vi "Main.vi"(11 "Module Admin":refnum<class "Delacor_lib_QMH_Module Admin.lvclass">) -> ()   [LabVIEW 2021, in "User Interface.lvlib"]
doc: "This template is based off of the Queued Message Handler design pattern and the Queued Message Handler project template that ships with LabVIEW.\n\nThe main difference is that the queue is private to this module and communication between modules is performed via Broadcast and Request events.\n\nRequest events are wrapped in public API methods and are handled in the Event Handling Loop (EHL) of this VI. Any module can register for Broadcast events sent by this module. The EHL generates messages based on user interface actions.\n\nThe Message Handling Loop (MHL) processes messages generated by the EHL, or by other messages. The messages are string values, so new messages can be added easily to the Message Cases case structure in the MHL. Each message cluster can also provide an optional value for Message Data, which is a variant that can be converted to whatever message-specific data is required.\n_____\nBased on DQMH Project Template 6.1.0.94."
uses:
  User Interface.lvlib
  <vilib>/Delacor/Delacor QMH/Libraries/Module Admin_class/Delacor_lib_QMH_Module Admin.lvclass
  Module Data--cluster.ctl
  <vilib>/Delacor/Delacor QMH/Libraries/Message Queue_class/Delacor_lib_QMH_Message Queue.lvclass/Delacor_lib_QMH_Message Queue.ctl
  Stop Argument--cluster.ctl
  <vilib>/Delacor/Delacor QMH/Libraries/Module Admin_class/Delacor_lib_QMH_Module Admin.lvclass/Delacor_lib_QMH_Module Admin.ctl
  REQ UI Title Argument--cluster.ctl
  <vilib>/Utility/miscctls.llb/LVPointTypeDef.ctl
  VI Name.ctl
  <vilib>/Delacor/Delacor QMH/Libraries/Message Queue_class/Delacor_lib_QMH_Enqueue Message (Single).vi
  <vilib>/Delacor/Delacor QMH/Libraries/Module Admin_class/Delacor_lib_QMH_Get External Launch.vi
  <vilib>/Utility/error.llb/Error Cluster From Error Code.vi
  <vilib>/ErrorRing/Error Ring.xnode
  <vilib>/Delacor/Delacor QMH/Libraries/Message Queue_class/Delacor_lib_QMH_Message Queue.lvclass
  Database/Database.lvlib
  CAN/CAN.lvlib
  DAQ Hardware/DAQ Hardware.lvlib
  DAQ IO/DAQ IO.lvlib
  ARINC/ARINC.lvlib
  DC PWS/DC PWS.lvlib
  DMM/DMM.lvlib
  Func Generator/Func Generator.lvlib
  Oscilloscope/Oscilloscope.lvlib
  S-Matrix/S-Matrix.lvlib
  Environment Chamber/Environment Chamber.lvlib
  CVT/CVT.lvlib
panel:
  out "Top Label":string="MAINTENANCE"
  out "Time":string="Sat  8/3/2019  8:10:44 PM"
  out "error out":errorcluster
  out "Status":string
  in  "Simulate MHL Error":bool
  in  "Simulate EHL Error":bool
  # "Other QMH Modules communicate with this Module via its Public API (wrappers for its Request Events).\n\nThis Module communicates with other Modules via its Broadcast Events.\nAny module that wants to get these messages, just registers for this module's Broadcast events."
  # "This template is for the Delacor Modified Queued Message Handler design pattern.\n\nSee the block diagram for more information on how to use this template."
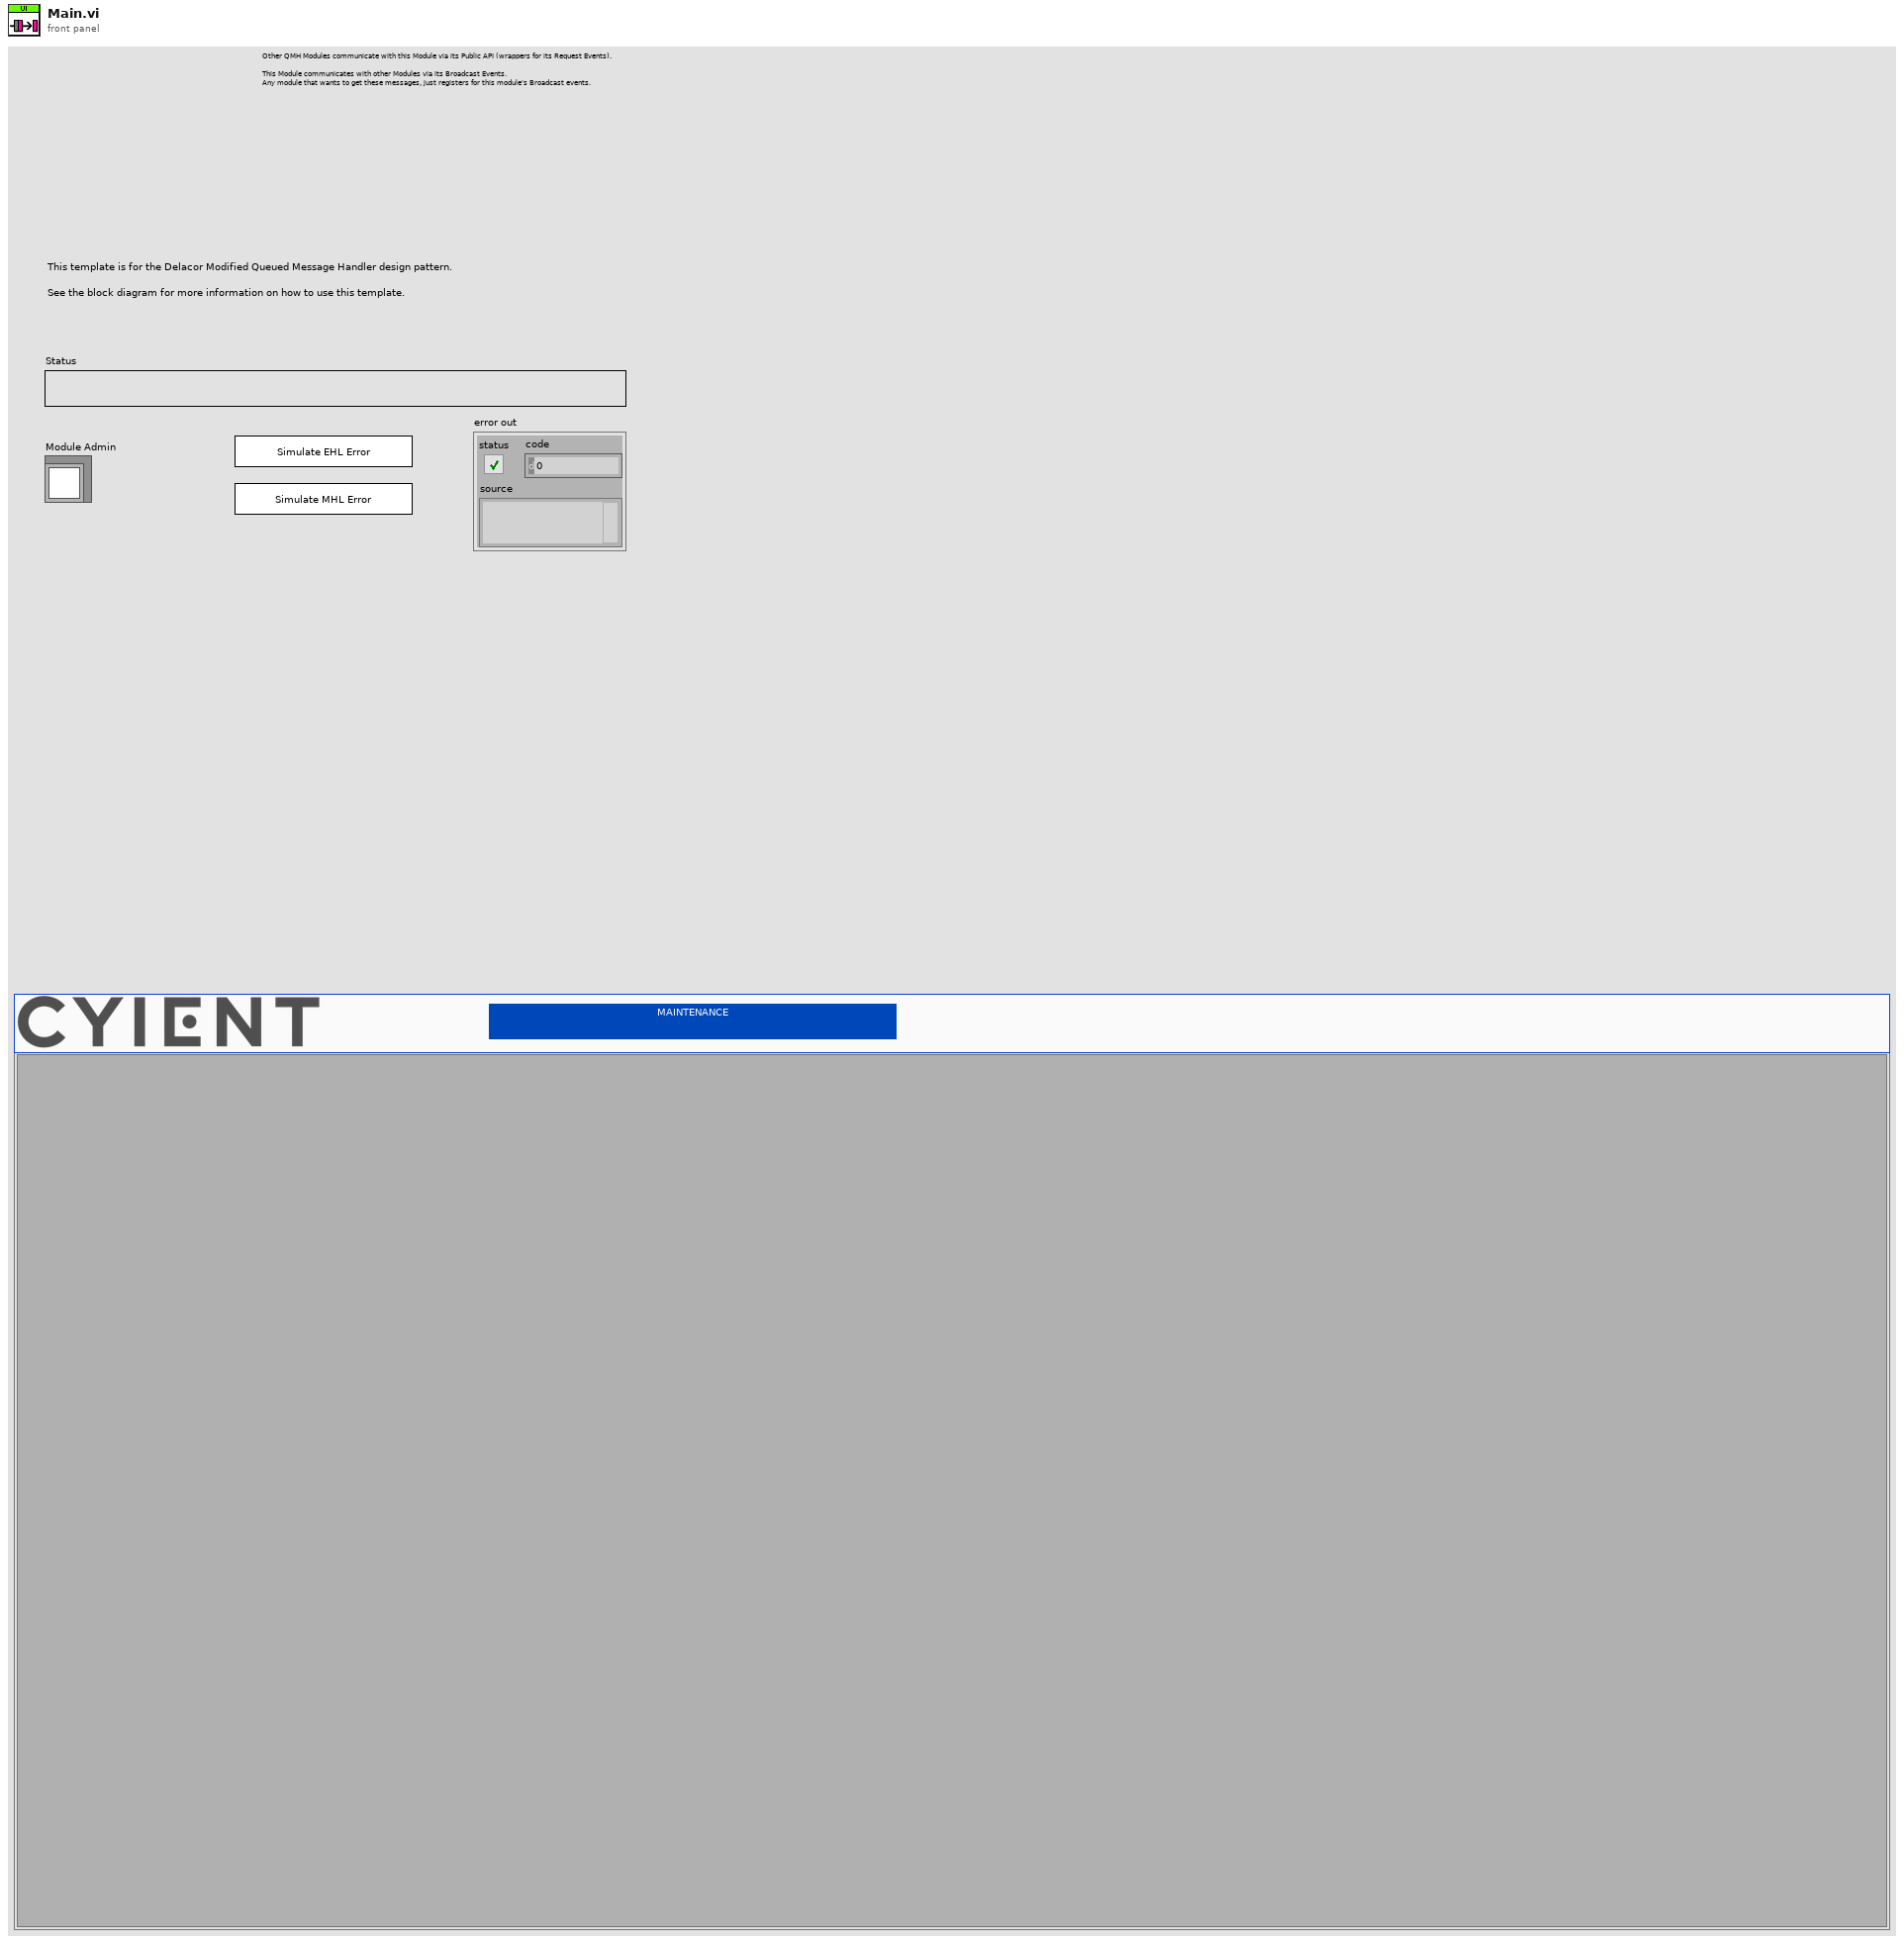
[diagram p1: front panel]
types:
  T1 = typedef "User Interface.lvlib/Request Events--cluster.ctl" = cluster{"Stop Module":refnum<user-event>, "Show Panel":refnum<user-event>, "Hide Panel":refnum<user-event>, "Get Module Execution Status":refnum<user-event>, "Show Diagram":refnum<user-event>, "REQ UI Title":refnum<user-event>}
  T2 = typedef "User Interface.lvlib/Module Data--cluster.ctl" = cluster{"Status":string}
  T3 = enum32{"invalid lock state", "Not Locked", "Locked (No Password)", "Password-protected"}
  T4 = typedef "User Interface.lvlib/Stop Argument--cluster.ctl" = cluster{"Origin":string, "Exit via Stop Module Req?":bool, "Wait for Module to stop?":bool}
  T5 = typedef "User Interface.lvlib/REQ UI Title Argument--cluster.ctl" = cluster{"UI Title":string}
  T6 = typedef "LVPointTypeDef.ctl" = cluster{"Horizontal":i16, "Vertical":i16}
  T7 = enum32{"Invalid", "Standard", "Closed", "Hidden", "Minimized", "Maximized"}
  T8 = typedef "User Interface.lvlib/VI Name.ctl" = enum16{"Dashboard", "Maintenance", "Recipe", "Inst Configuration", "Testing", "Report"}
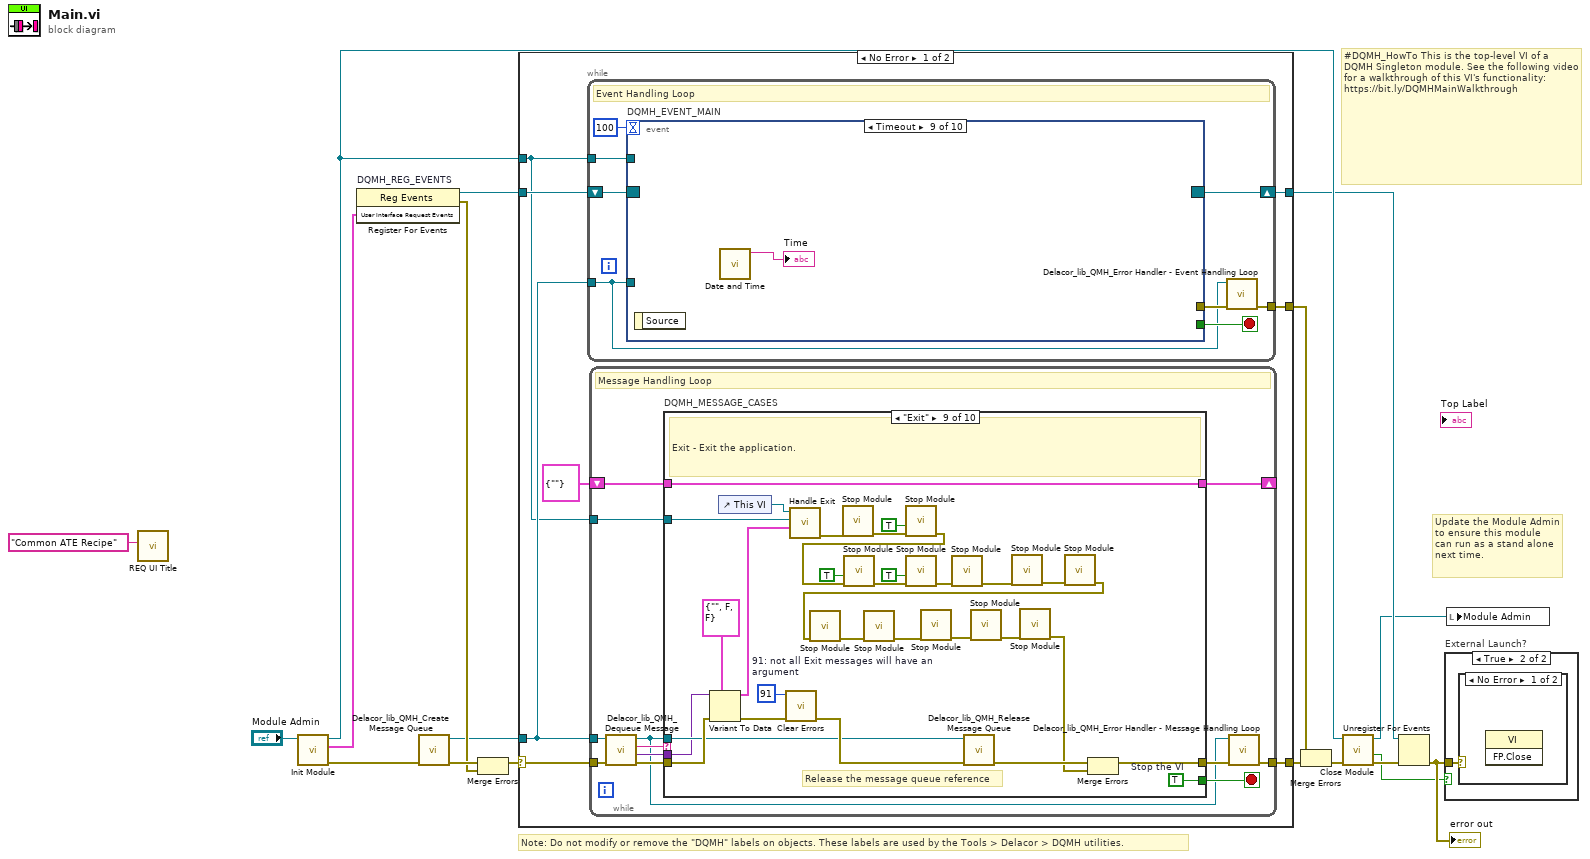
[diagram p0: block diagram]
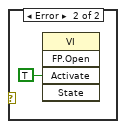
[diagram p3: hidden frame]
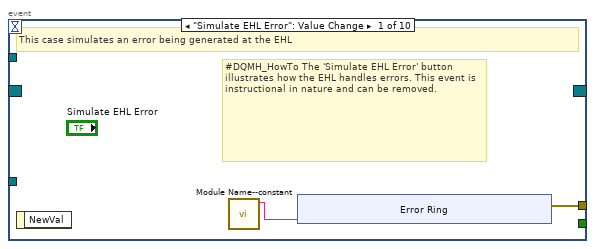
[diagram p4: hidden frame]
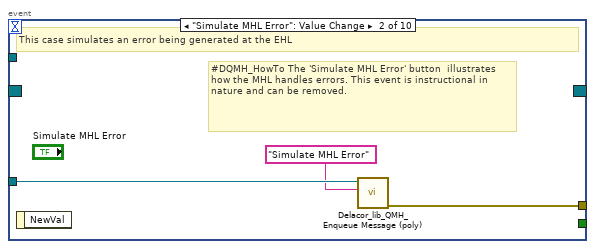
[diagram p5: hidden frame]
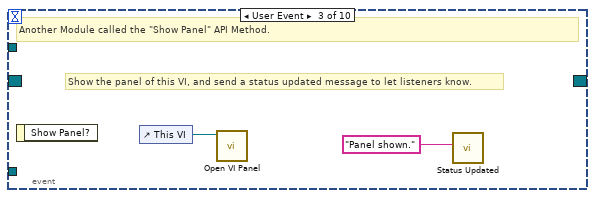
[diagram p6: hidden frame]
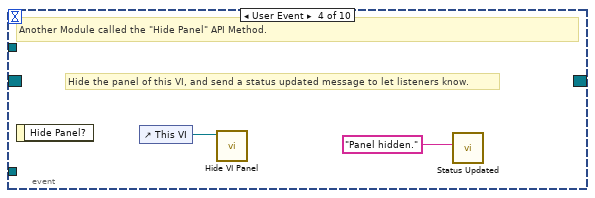
[diagram p7: hidden frame]
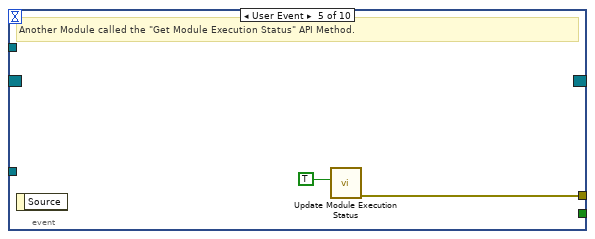
[diagram p8: hidden frame]
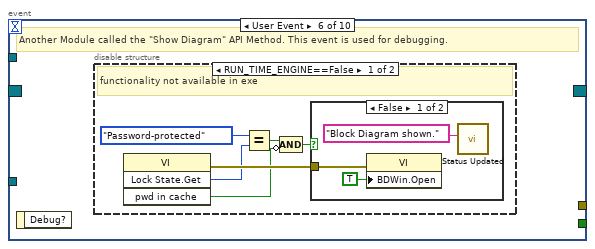
[diagram p9: hidden frame]
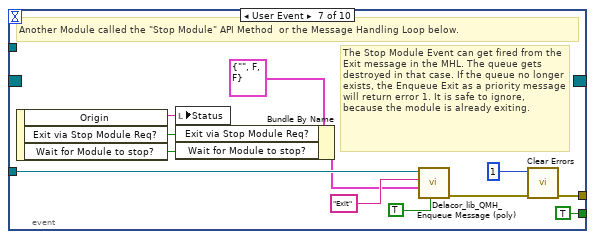
[diagram p12: hidden frame]
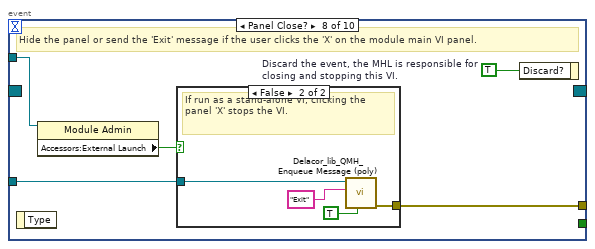
[diagram p13: hidden frame]
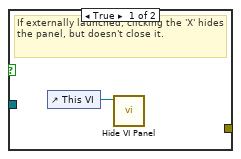
[diagram p14: hidden frame]
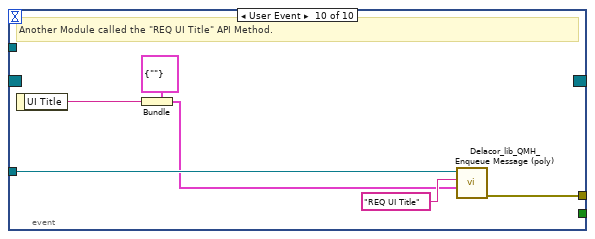
[diagram p15: hidden frame]
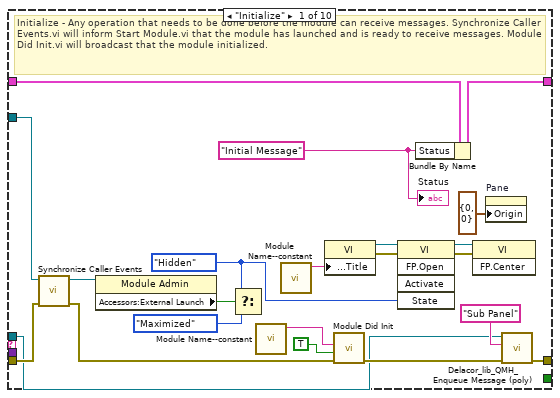
[diagram p16: hidden frame]
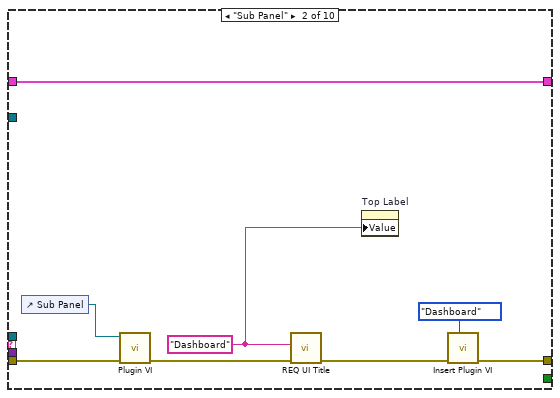
[diagram p17: hidden frame]
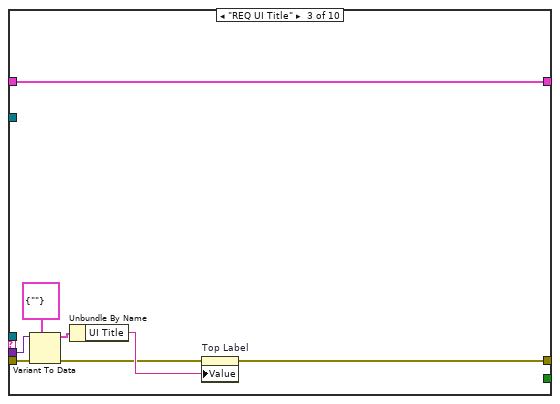
[diagram p18: hidden frame]
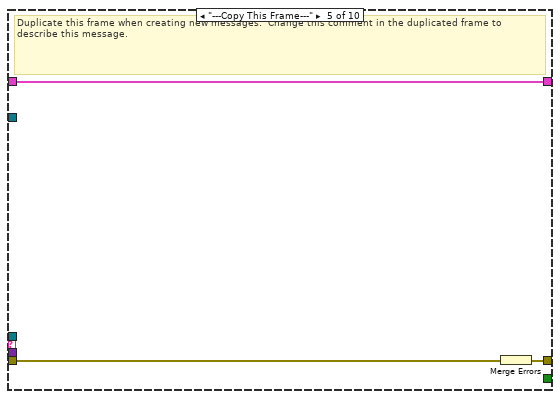
[diagram p20: hidden frame]
diagram:
  # "#DQMH_HowTo This is the top-level VI of a DQMH Singleton module. See the following video for a walkthrough of this VI's functionality: https://bit.ly/DQMHMainWalkthrough"
  # "Note: Do not modify or remove the \"DQMH\" labels on objects. These labels are used by the Tools > Delacor > DQMH utilities."
  # "Update the Module Admin to ensure this module can run as a stand alone next time."
  n1 = call "REQ UI Title.vi"("UI Title"="Common ATE Recipe") -> ()  [unwired: 10 in, 1 out]
  n2 = call "Init Module.vi"("Singleton Module Admin in"="Module Admin") -> ("error out"=w17:errorcluster, "User Interface Request Events"=w6:T1, "Singleton Module Admin out"=w9:refnum<class "Delacor_lib_QMH_Module Admin.lvclass">)  [unwired: 8 in]
  n3 = register-events "DQMH_REG_EVENTS"(w6) -> (reference out=w7:refnum<event-registration>, error out=w10:errorcluster)  [unwired: 2 in]
  n4 = call <vilib>:"Delacor_lib_QMH_Create Message Queue.vi"("error in"=w17) -> ("error out"=w12:errorcluster, "Message Queue"=w5:refnum<class "Delacor_lib_QMH_Message Queue.lvclass">)  [unwired: 9 in]
  n5 = Merge Errors(w12, w10) -> (w11:errorcluster)
  n6 = case shown="No Error" w11 {
    selector: w11 -> [w24 w222]
    tunnel: [w26 w221] -> w18
    tunnel: [w23 w227] -> w8
    tunnel: w7 -> [w21 w227]
    tunnel: w5 -> [w20 w220]
    tunnel: [w25 _] -> w15
    tunnel: w9 -> [w19 w223]
    frame No Error {
      n7 = while {
        tunnel: w20 -> [w28]
        shift-right: [w31] -> w23
        shift-left: w21 -> [w32]
        tunnel: [w33] -> w25
        tunnel: w19 -> [w29]
        stop <- w30 stop-if-true
        # "Event Handling Loop"
        n8 = event "DQMH_EVENT_MAIN" shown="[8] Timeout" {
          selector: w32 -> [_ _ _ _ _ _ _ _ _ _]
          dyn-events: [_ _ _ _ _ _ _ _ _ _] -> w31
          timeout: 100 -> [_ _ _ _ _ _ _ _ _ _]
          tunnel: [_ _ _ _ _ _ TRUE ("Discard?") _ _ _] -> w30
          tunnel: w28 -> [_ w45 _ _ _ _ w69 w76 _ w90]
          tunnel: [w36 w46 _ _ w52 _ w72 w78 _ w85] -> w34
          tunnel: w29 -> [_ _ _ _ _ _ _ w75 _ _]
          event "Simulate EHL Error": Value Change {
            # "#DQMH_HowTo The 'Simulate EHL Error' button  illustrates how the EHL handles errors. This event is instructional in nature and can be removed."
            # "This case simulates an error being generated at the EHL"
            n9 = event-data() -> ()  [unwired: 1 in, 1 out]
            n10 = call "Module Name--constant.vi"() -> ("Module Name"=w35:string)  [unwired: 11 in]
            n11 = xnode "Error Ring"("parameter 0"=w35) -> ("error out"=w36:errorcluster)
          }
          event "Simulate MHL Error": Value Change {
            # "#DQMH_HowTo The 'Simulate MHL Error' button  illustrates how the MHL handles errors. This event is instructional in nature and can be removed."
            # "This case simulates an error being generated at the EHL"
            n12 = event-data() -> ()  [unwired: 1 in, 1 out]
            n13 = call-poly <vilib>:"Delacor_lib_QMH_Enqueue Message (poly).vi"("Message"="Simulate MHL Error", "Message Queue in"=w45) -> ("error out"=w46:errorcluster)  [unwired: 8 in, 1 out]
          }
          event User Event {
            # "Show the panel of this VI, and send a status updated message to let listeners know."
            # "Another Module called the \"Show Panel\" API Method."
            n14 = event-data() -> ()  [unwired: 1 in, 1 out]
            n15 = control-ref of="This VI"() -> (w48:refnum<vi>)
            n16 = call "Open VI Panel.vi"("VI"=w48) -> ()  [unwired: 10 in, 1 out]
            n17 = call "Status Updated.vi"("Status"="Panel shown." ("format string")) -> ()  [unwired: 10 in, 1 out]
          }
          event User Event {
            # "Hide the panel of this VI, and send a status updated message to let listeners know."
            # "Another Module called the \"Hide Panel\" API Method."
            n18 = event-data() -> ()  [unwired: 1 in, 1 out]
            n19 = control-ref of="This VI"() -> (w50:refnum<vi>)
            n20 = call "Hide VI Panel.vi"("VI"=w50) -> ()  [unwired: 10 in, 1 out]
            n21 = call "Status Updated.vi"("Status"="Panel hidden." ("format string")) -> ()  [unwired: 10 in, 1 out]
          }
          event User Event {
            # "Another Module called the \"Get Module Execution Status\" API Method."
            n22 = event-data() -> ()  [unwired: 1 in, 1 out]
            n23 = call "Update Module Execution Status.vi"("Running?"=TRUE) -> ("error out"=w52:errorcluster)  [unwired: 10 in]
          }
          event User Event {
            # "Another Module called the \"Show Diagram\" API Method. This event is used for debugging."
            n24 = event-data() -> ()  [unwired: 1 in, 1 out]
            n25 = disable-structure shown="RUN_TIME_ENGINE==False" {
              frame condition #0 (active) {
                # "functionality not available in exe"
                n26 = invoke class="VI" method="Lock State.Get"() -> (error out=w58:errorcluster, "Get Lock State"=w57:T3, "pwd in cache"=w54:bool)  [unwired: 4 in, 1 out]
                n27 = Equal?(x=T3."Password-protected", y=w57) -> (x = y?=w55:bool)
                n28 = Compound Arithmetic op=AND(w55, invert w54) -> (w53:bool)
                n29 = case shown="False" w53 {
                  tunnel: w58 -> [w61 _]
                  frame False {
                    n30 = property class="VI"(error in=w61, "BDWin.Open"=TRUE ("Block Diagram Window:Open")) -> ()  [unwired: 1 in, 2 out]
                    n31 = call "Status Updated.vi"("Status"="Block Diagram shown." ("format string")) -> ()  [unwired: 10 in, 1 out]
                  }
                  frame True {
                    # "Password-protected VI, and the password is not in the cache. Do not show the diagram."
                  }
                }
              }
              frame condition #1 {
              }
            }
          }
          event User Event {
            # "The Stop Module Event can get fired from the Exit message in the MHL. The queue gets destroyed in that case. If the queue no longer exists, the Enqueue Exit as a priority message will return error 1. It is safe to ignore, because the module is already exiting."
            # "Another Module called the \"Stop Module\" API Method  or the Message Handling Loop below."
            n32 = event-data() -> ("Origin"=w68:string, "Exit via Stop Module Req?"=w64:bool, "Wait for Module to stop?"=w63:bool)  [unwired: 1 in]
            n33 = local write "Status"(w68) -> ()
            n34 = Bundle By Name(cluster=T4 {"Origin"="", "Exit via Stop Module Req?"=FALSE, "Wait for Module to stop?"=FALSE} ("Stop Argument"), "Exit via Stop Module Req?"=w64, "Wait for Module to stop?"=w63) -> (w62:T4)
            n35 = call-poly <vilib>:"Delacor_lib_QMH_Enqueue Message (poly).vi"("Priority Message? (F)"=TRUE, "Message Data"=w62, "Message"="Exit", "Message Queue in"=w69) -> ("error out"=w73:errorcluster)  [unwired: 6 in, 1 out]
            n36 = call <vilib>:"Clear Errors.vi"("error in (no error)"=w73, "specific error code to clear (0: all)"=1) -> ("error out"=w72:errorcluster)  [unwired: 4 in, 1 out]
          }
          event Panel Close? {
            w77 = TRUE  # Discard the event, the MHL is responsible for closing and stopping this VI.
            # "Hide the panel or send the 'Exit' message if the user clicks the 'X' on the module main VI panel."
            n37 = event-data() -> ()  [unwired: 1 in, 1 out]
            n38 = property class="Module Admin"(reference=w75) -> ("Accessors:External Launch"=w74:bool)  [unwired: 1 in, 2 out]
            n39 = case shown="False" w74 {
              tunnel: w76 -> [_ w82]
              tunnel: [_ w83] -> w78
              frame True {
                # "If externally launched, clicking the 'X' hides the panel, but doesn't close it."
                n40 = control-ref of="This VI"() -> (w79:refnum<vi>)
                n41 = call "Hide VI Panel.vi"("VI"=w79) -> ()  [unwired: 10 in, 1 out]
              }
              frame False {
                # "If run as a stand-alone VI, clicking the panel 'X' stops the VI."
                n42 = call-poly <vilib>:"Delacor_lib_QMH_Enqueue Message (poly).vi"("Priority Message? (F)"=TRUE, "Message"="Exit", "Message Queue in"=w82) -> ("error out"=w83:errorcluster)  [unwired: 7 in, 1 out]
              }
            }
            n43 = event-data("Discard?"=w77) -> ()  [unwired: 1 in, 1 out]
          }
          event Timeout {
            n44 = event-data() -> ()  [unwired: 1 in, 1 out]
            n45 = call "Date and Time.vi"() -> ("Current Time"=→"Time":string)  [unwired: 11 in]
          }
          event User Event {
            # "Another Module called the \"REQ UI Title\" API Method."
            n46 = event-data() -> ("UI Title"=w86:string)  [unwired: 1 in]
            n47 = Bundle(cluster=T5 {"UI Title"=""} ("REQ UI Title Argument"), "UI Title"=w86) -> (w87:T5)
            n48 = call-poly <vilib>:"Delacor_lib_QMH_Enqueue Message (poly).vi"("Message Data"=w87, "Message"="REQ UI Title", "Message Queue in"=w90) -> ("error out"=w85:errorcluster)  [unwired: 7 in, 1 out]
          }
        }
        n49 = call-dynamic "Delacor_lib_QMH_Error Handler - Event Handling Loop.vi"("error in"=w34, "Message Queue in"=w28) -> ("dup error in"=w33:errorcluster)  [unwired: 8 in, 1 out]
      }
      n50 = while {
        tunnel: w20 -> [w93]
        shift-right: [w97] -> _
        shift-left: T2 {"Status"=""} ("Data Cluster") -> [w98]
        tunnel: w24 -> [w101]
        tunnel: [w99] -> w26
        tunnel: w19 -> [w91]
        stop <- w96 stop-if-true
        # "Message Handling Loop"
        n51 = call-dynamic "Delacor_lib_QMH_Dequeue Message.vi"("error in"=w101, "Message Queue in"=w93) -> ("error out"=w100:errorcluster, "Message Data"=w94:variant, "Message"=w95:string, "Message Queue out"=w92:refnum<class "Delacor_lib_QMH_Message Queue.lvclass">)  [unwired: 6 in]
        n52 = case "DQMH_MESSAGE_CASES" shown="\"Exit\"" w95 {
          selector: w95 -> [_ _ _ _ _ _ _ _ _ w207]
          tunnel: w92 -> [w105 _ _ _ _ _ _ w162 w200 _]
          tunnel: w100 -> [w122 w130 w140 w142 w145 w147 w152 w169 w205 w209]
          tunnel: [w106 w129 w133 w142 w144 w147 w151 w165 w202 w210] -> w102
          tunnel: w98 -> [w115 w132 w139 w141 w143 w146 w149 w164 w199 w208]
          tunnel: [w114 w132 w139 w141 w143 w146 w149 w164 w199 w208] -> w97
          tunnel: [_ _ _ _ _ _ _ _ w198 _] -> w96
          tunnel: w94 -> [_ _ w138 _ _ _ _ w163 w197 _]
          tunnel: w91 -> [w116 _ _ _ _ _ _ w161 w192 _]
          frame "Initialize" {
            w110 = "Initial Message" ("Initial Message")
            w103 = T7."Hidden" ("State")
            # "Initialize - Any operation that needs to be done before the module can receive messages. Synchronize Caller Events.vi will inform Start Module.vi that the module has launched and is ready to receive messages. Module Did Init.vi will broadcast that the module initialized."
            n53 = call "Synchronize Caller Events.vi"("error in (no error)"=w122, "Singleton Module Admin in"=w116) -> ("error out"=w121:errorcluster, "Singleton Module Admin out"=w111:refnum<class "Delacor_lib_QMH_Module Admin.lvclass">)  [unwired: 8 in]
            n54 = property class="Module Admin"(reference=w111) -> ("Accessors:External Launch"=w117:bool)  [unwired: 1 in, 2 out]
            n55 = Select(t=w103, s=w117, f=T7."Maximized" ("State")) -> ()  [unwired: 1 out]
            n56 = call "Module Name--constant.vi"() -> ("Module Name"=w112:string)  [unwired: 11 in]
            n57 = call "Module Name--constant.vi"() -> ("Module Name"=w120:string)  [unwired: 11 in]
            n58 = property class="VI"("Front Panel.Title"=w120) -> (reference out=w119:refnum<vi>, error out=w124:errorcluster)  [unwired: 2 in]
            n59 = call "Module Did Init.vi"("error in (no error)"=w121, "Initialized?"=TRUE, "Origin"=w112) -> ("error out"=w107:errorcluster)  [unwired: 8 in]
            n60 = invoke class="VI" method="FP.Open"(reference=w119, error in=w124, "State"=w103) -> (reference out=w118:refnum<vi>, error out=w123:errorcluster)  [unwired: 2 in, 3 out]
            n61 = Bundle By Name(cluster=w115, "Status"=w110) -> (w114:T2)
            n62 = invoke class="VI" method="FP.Center"(reference=w118, error in=w123) -> ()  [unwired: 1 in, 3 out]
            n63 = property on="Pane" class="Pane"("Origin"=T6 {"Horizontal"=0, "Vertical"=0}) -> ()  [unwired: 2 in, 2 out]
            n64 = call-poly <vilib>:"Delacor_lib_QMH_Enqueue Message (poly).vi"("error in"=w107, "Message"="Sub Panel", "Message Queue in"=w105) -> ("error out"=w106:errorcluster)  [unwired: 7 in, 1 out]
            "Status" <- w110
          }
          frame "Sub Panel" {
            w125 = "Dashboard" ("ATE Title")
            n65 = control-ref of="Sub Panel"() -> (w131:refnum<vi>)
            n66 = call "Plugin VI.vi"("error in (no error)"=w130, "Sub Panel"=w131) -> ("error out"=w127:errorcluster)  [unwired: 9 in]
            n67 = call "REQ UI Title.vi"("error in"=w127, "UI Title"=w125) -> ("error out"=w126:errorcluster)  [unwired: 9 in]
            n68 = property on="Top Label" class="Str"("Value"=w125) -> ()  [unwired: 2 in, 2 out]
            n69 = call "Insert Plugin VI.vi"("VI Name"=VI_Name."Dashboard", "error in (no error)"=w126) -> ("error out"=w129:errorcluster)  [unwired: 9 in]
          }
          frame "REQ UI Title" {
            n70 = Variant To Data(error in=w140, type=T5 {"UI Title"=""} ("REQ UI Title Argument"), Variant=w138) -> (data=w136:T5, error out=w134:errorcluster)
            n71 = Unbundle By Name(w136) -> ("UI Title"=w135:string)
            n72 = property on="Top Label" class="Str"(error in=w134, "Value"=w135) -> (error out=w133:errorcluster)  [unwired: 1 in, 1 out]
          }
          frame "---Module Specific---" {
            # "Separator -- The following cases handle messages specific to this Module."
          }
          frame "---Copy This Frame---" {
            # "Duplicate this frame when creating new messages.  Change this comment in the duplicated frame to describe this message."
            n73 = Merge Errors(w145) -> (w144:errorcluster)
          }
          frame "---Exit and Error Handling---" {
            # "Separator - The following cases handle errors and exit messages."
          }
          frame "Simulate MHL Error" {
            # "#DQMH_HowTo The 'Simulate MHL Error' button  illustrates how the MHL handles errors. This event is instructional in nature and can be removed."
            # "Simulate an error occurring at the MHL"
            n74 = call "Module Name--constant.vi"() -> ("Module Name"=w148:string)  [unwired: 11 in]
            n75 = xnode "Error Ring"("parameter 0"=w148) -> ("error out"=w150:errorcluster)
            n76 = Merge Errors(w152, w150) -> (w151:errorcluster)
          }
          frame "Error" {
            # "#CodeRecommended - If you ever change the name of this \"Error\" message, you'll need to update the name in the Check Loop Error.vi as well."
            # "#CodeRecommended - If the module is running in standalone mode (External Launch = FALSE), this code will pop up an error dialog and call the 'Exit' message if an error occurs. Add more fine-grained error handling here."
            # "Error - Check the error message data and respond accordingly. This message is sent by the \"Error Handler\" VIs at the end of each loop in this application."
            n77 = property class="Module Admin"(reference=w161) -> ("Accessors:External Launch"=w160:bool)  [unwired: 1 in, 2 out]
            n78 = Variant To Data(error in=w169, type=errorcluster {"status"=FALSE, "code"=0, "source"=""} ("error constant"), Variant=w163) -> (data=w170:errorcluster, error out=w167:errorcluster)
            n79 = call "Error Reported.vi"("Error"=w170) -> ()  [unwired: 10 in, 1 out]
            n80 = case shown="False" w160 {
              tunnel: [w175 _] -> w166
              tunnel: w162 -> [w173 _]
              tunnel: w170 -> [w174 _]
              frame False {
                # "If the module is running standalone, then pop up an error dialog and call the \"Exit\" message."
                n81 = call <vilib>:"Simple Error Handler.vi"("error in (no error)"=w174) -> ()  [unwired: 4 in, 5 out]
                n82 = call-poly <vilib>:"Delacor_lib_QMH_Enqueue Message (poly).vi"("Priority Message? (F)"=TRUE, "Message"="Exit", "Message Queue in"=w173) -> ("error out"=w175:errorcluster)  [unwired: 7 in, 1 out]
              }
              frame True {
                # "If the module was launched externally, calling the Error Reported broadcast VI is the only action performed by the \"Error\" message. The module's caller can then process the error appropriately."
              }
            }
            n83 = Merge Errors(w167, w166) -> (w165:errorcluster)
            n84 = local write "error out"(w165) -> ()
          }
          frame "Exit" {
            w196 = 91  # 91: not all Exit messages will have an argument
            w198 = TRUE  # Stop the VI
            # "Release the message queue reference"
            # "Exit - Exit the application."
            n85 = Variant To Data(error in=w205, type=T4 {"Origin"="", "Exit via Stop Module Req?"=FALSE, "Wait for Module to stop?"=FALSE} ("Stop Argument"), Variant=w197) -> (data=w194:T4, error out=w201:errorcluster)
            n86 = control-ref of="This VI"() -> (w193:refnum<vi>)
            n87 = call <vilib>:"Clear Errors.vi"("error in (no error)"=w201, "specific error code to clear (0: all)"=w196) -> ("error out"=w204:errorcluster)  [unwired: 4 in, 1 out]
            n88 = call "Handle Exit.vi"("Stop Argument"=w194, "Admin in"=w192, "VI reference"=w193) -> ("error out"=w188:errorcluster)  [unwired: 7 in, 1 out]
            n89 = call "Stop Module.vi"("error in"=w188) -> ("error out"=w191:errorcluster)  [unwired: 10 in]
            n90 = call "Stop Module.vi"("error in"=w191, "Wait for Module to Stop? (F)"=TRUE) -> ("error out"=w183:errorcluster)  [unwired: 9 in]
            n91 = call "Stop Module.vi"("error in"=w183, "Wait for Module to Stop? (F)"=TRUE) -> ("error out"=w184:errorcluster)  [unwired: 9 in]
            n92 = call "Stop Module.vi"("error in"=w184, "Wait for Module to Stop? (F)"=TRUE) -> ("error out"=w182:errorcluster)  [unwired: 9 in]
            n93 = call "Stop Module.vi"("error in"=w182) -> ("error out"=w187:errorcluster)  [unwired: 10 in]
            n94 = call-dynamic "Delacor_lib_QMH_Release Message Queue.vi"("error in"=w204, "Message Queue"=w200) -> ("error out"=w203:errorcluster)  [unwired: 9 in]
            n95 = call "Stop Module.vi"("error in"=w187) -> ("error out"=w181:errorcluster)  [unwired: 10 in]
            n96 = call "Stop Module.vi"("error in"=w181) -> ("error out"=w180:errorcluster)  [unwired: 10 in]
            n97 = call "Stop Module.vi"("error in"=w180) -> ("error out"=w185:errorcluster)  [unwired: 10 in]
            n98 = call "Stop Module.vi"("error in"=w185) -> ("error out"=w186:errorcluster)  [unwired: 10 in]
            n99 = call "Stop Module.vi"("error in"=w186) -> ("error out"=w179:errorcluster)  [unwired: 10 in]
            n100 = call "Stop Module.vi"("error in"=w179) -> ("error out"=w177:errorcluster)  [unwired: 10 in]
            n101 = call "Stop Module.vi"("error in"=w177) -> ("error out"=w176:errorcluster)  [unwired: 10 in]
            n102 = Merge Errors(w203, w176) -> (w202:errorcluster)
          }
          frame Default {
            # "'Default' case only runs if there is a message that isn't defined in any of the other cases.  Output a programming error."
            n103 = call "Module Name--constant.vi"() -> ("Module Name"=w206:string)  [unwired: 11 in]
            n104 = xnode "Error Ring"("parameter 0"=w207, "parameter 1"=w206) -> ("error out"=w211:errorcluster)
            n105 = Merge Errors(w209, w211) -> (w210:errorcluster)
          }
        }
        n106 = call-dynamic "Delacor_lib_QMH_Error Handler - Message Handling Loop.vi"("error in"=w102, "Message Queue in"=w92) -> ("dup error in"=w99:errorcluster)  [unwired: 8 in, 1 out]
      }
    }
    frame Error {
      # "Synchronize Caller Events.vi will inform Start Module.vi that the module has launched and will let the code calling Start Module.vi register for broadcasts and would permit the caller receive the broadcast that an error occurred at launch time."
      n107 = call-dynamic "Delacor_lib_QMH_Release Message Queue.vi"("error in"=w222, "Message Queue"=w220) -> ("error out"=w221:errorcluster)  [unwired: 9 in]
      n108 = call "Synchronize Caller Events.vi"("Singleton Module Admin in"=w223) -> ("error out"=w228:errorcluster)  [unwired: 9 in, 1 out]
      n109 = call "Module Name--constant.vi"() -> ("Module Name"=w226:string)  [unwired: 11 in]
      n110 = Format Into String(format string="An error occurred during initialization. %s is no longer running.", w226) -> (resulting string=w224:string)  [unwired: 2 in, 1 out]
      n111 = Merge Errors(w221, w228) -> (w229:errorcluster)
      n112 = call "Error Reported.vi"("Additional Information"=w224, "Error"=w229) -> ()  [unwired: 9 in, 1 out]
    }
  }
  n113 = Merge Errors(w15, w18) -> (w14:errorcluster)
  n114 = call "Close Module.vi"("error in (no error)"=w14, "Module Admin in"=w9) -> ("error out"=w16:errorcluster, "External Launch"=w2:bool, "Module Admin out"=w3:refnum<class "Delacor_lib_QMH_Module Admin.lvclass">)  [unwired: 7 in]
  n115 = Unregister For Events(event registration refnum=w8, error in=w16) -> (error out=w13:errorcluster)
  "error out" <- w13
  n116 = case "External Launch?" shown="True" w2 {
    tunnel: w13 -> [_ w230]
    frame False {
    }
    frame True {
      n117 = case shown="No Error" w230 {
        frame No Error {
          n118 = invoke class="VI" method="FP.Close"() -> ()  [unwired: 3 in, 3 out]
        }
        frame Error {
          n119 = invoke class="VI" method="FP.Open"("Activate"=TRUE ("Activate?")) -> ()  [unwired: 4 in, 5 out]
        }
      }
    }
  }
  n120 = local write "Module Admin"(w3) -> ()
